vi "Determine data type and ROI ID.vi"(11 "Dataset path":refnum<vi>) -> (1 "Valid path":bool, 2 "Functional data type":T2, 3 "ROI ID Enum":T1)   [LabVIEW 2017]
uses:
  Typedefs/Functional data family.ctl
  Typedefs/ROI ID Enum.ctl
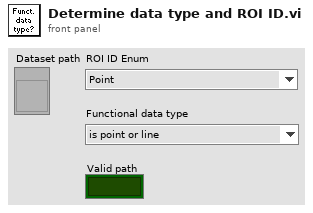
[diagram p1: front panel]
types:
  T1 = typedef "ROI ID Enum.ctl" = enum16{"Point", "MiniScan", "Comp. MiniScan", "Rectangle", "Comp. volume", "Arb. plane point"}
  T2 = typedef "Functional data family.ctl" = enum16{"is point or line", "is surface or volume"}
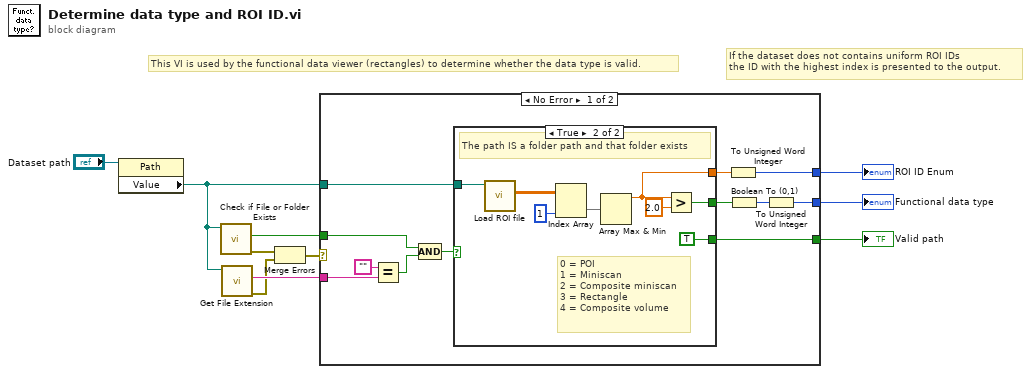
[diagram p0: block diagram]
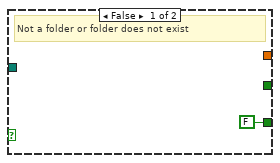
[diagram p2: hidden frame]
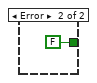
[diagram p3: hidden frame]
diagram:
  # "If the dataset does not contains uniform ROI IDs\nthe ID with the highest index is presented to the output."
  # "This VI is used by the functional data viewer (rectangles) to determine whether the data type is valid."
  n1 = property class="Path"(reference="Dataset path") -> ("Value"=w7:path)  [unwired: 1 in, 2 out]
  n2 = call <vilib>:"Check if File or Folder Exists.vi"("path"=w7) -> ("error out"=w3:errorcluster, "file or folder exists?"=w4:bool)  [unwired: 8 in, 1 out]
  n3 = call <vilib>:"Get File Extension.vi"("file"=w7) -> ("error out"=w2:errorcluster, "lowercase file extension"=w5:string)  [unwired: 6 in, 3 out]
  n4 = Merge Errors(w3, w2) -> (w1:errorcluster)
  n5 = case shown="No Error" w1 {
    tunnel: [w22 _] -> w10
    tunnel: [w20 _] -> w9
    tunnel: [w17 FALSE] -> w8
    tunnel: w7 -> [w16 _]
    tunnel: w5 -> [w14 _]
    tunnel: w4 -> [w11 _]
    frame No Error {
      n6 = Equal?(x="", y=w14) -> (x = y?=w12:bool)
      n7 = Compound Arithmetic op=AND(w11, w12) -> (w15:bool)
      n8 = case shown="True" w15 {
        tunnel: w16 -> [_ w31]
        tunnel: [_ w26] -> w18
        tunnel: [FALSE TRUE] -> w17
        tunnel: [_ w24] -> w21
        frame False {
          # "Not a folder or folder does not exist"
        }
        frame True {
          # "0 = POI\t \n1 = Miniscan\n2 = Composite miniscan\n3 = Rectangle\n4 = Composite volume"
          # "The path IS a folder path and that folder exists"
          n9 = call "Load ROI file.vi"("Experiment data folder path"=w31) -> ("ROI Data (header removed)"=w30:dbl[][])  [unwired: 7 in, 3 out]
          n10 = Index Array(array=w30, index (col)=1 ("disabled index (col)")) -> (element=w28:dbl[])  [unwired: 1 in]
          n11 = Array Max & Min(array=w28) -> (max value=w24:dbl)  [unwired: 3 out]
          n12 = Greater?(x=w24, y=2.0) -> (0:w26:bool)
        }
      }
      n13 = To Unsigned Word Integer(number=w21) -> (unsigned 16bit integer=w22:u16)
      n14 = Boolean To (0,1)(Boolean=w18) -> (0, 1=w19:i16)
      n15 = To Unsigned Word Integer(number=w19) -> (unsigned 16bit integer=w20:u16)
    }
    frame Error {
    }
  }
  "Valid path" <- w8
  "Functional data type" <- w9
  "ROI ID Enum" <- w10
